vi "temperature_convert_K.vi"(4 "Data Keithley In":dbl[](array[numeric])) -> (1 "Data Keithley Out":dbl[](array[numeric]))   [LabVIEW 2011]
uses:
  <vilib>/express/express arith-compare/Formula/XNode/ExpressFormulaBlockNode.xnode
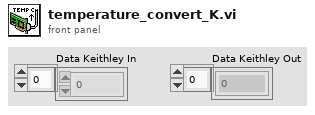
[diagram p1: front panel]
types:
  T1 = cluster{"Data Keithley In[0]":dbl, "Data Keithley In[1]":dbl, "Data Keithley In[2]":dbl, "Data Keithley In[3]":dbl, "Data Keithley In[4]":dbl, "Data Keithley In[5]":dbl, "Data Keithley In[6]":dbl, "Data Keithley In[7]":dbl, "Data Keithley In[8]":dbl}
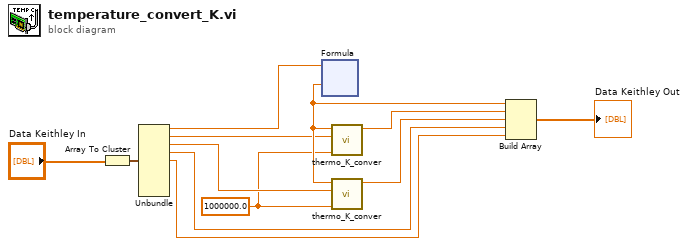
[diagram p0: block diagram]
diagram:
  w2 = 1000000.0 ("y")
  n1 = Array To Cluster(array="Data Keithley In") -> (cluster=w1:T1)
  n2 = Unbundle(w1) -> ("Data Keithley In[0]"=w3:dbl, "Data Keithley In[1]"=w4:dbl, "Data Keithley In[2]"=w5:dbl, "Data Keithley In[3]"=w10:dbl, "Data Keithley In[4]"=w7:dbl)  [unwired: 4 out]
  n3 = xnode ("Formula")("R"=w3) -> ("Result"=w6:dbl)  [unwired: 1 in, 1 out]
  n4 = call "thermo_K_conver.vi"("y"=w2, "Measurement Data[1]"=w4, "Measurement Data[0]"=w6) -> ("Result"=w8:dbl)  [unwired: 8 in]
  n5 = call "thermo_K_conver.vi"("y"=w2, "Measurement Data[1]"=w5, "Measurement Data[0]"=w6) -> ("Result"=w9:dbl)  [unwired: 8 in]
  n6 = Build Array(w6, w8, w9, w10, w7) -> (→"Data Keithley Out":dbl[])
